vi "About Dialog.vi"(9 "E-mail:":string="msira@cmil.cz", 10 "Maintainer:":string="Martin Šíra", 11 "Title":string="Filter function meter - WAC software bundle") -> ()   [LabVIEW 2020]
doc: "Shows application about dialog."
uses:
  <vilib>/Platform/browser.llb/Open URL in Default Browser (string).vi
  external libraries/varilib/varilib.lvlib
panel:
  in  "open web":bool
  out "copyright":string="author"
  in  "OK":bool
  out "address":string="Created in scope of the EPM project WAC.\nDistributed under the MIT license.\n\nAuthors:\n Martin Šíra, msira@cmi.cz\n \n For authors of the low level instrument drivers see\n readmes in the sourcecode."
  out "www:":string="http://www.tracepqm.cmi.cz\nhttps://github.com/smaslan/TWM"
  out "Version:":string
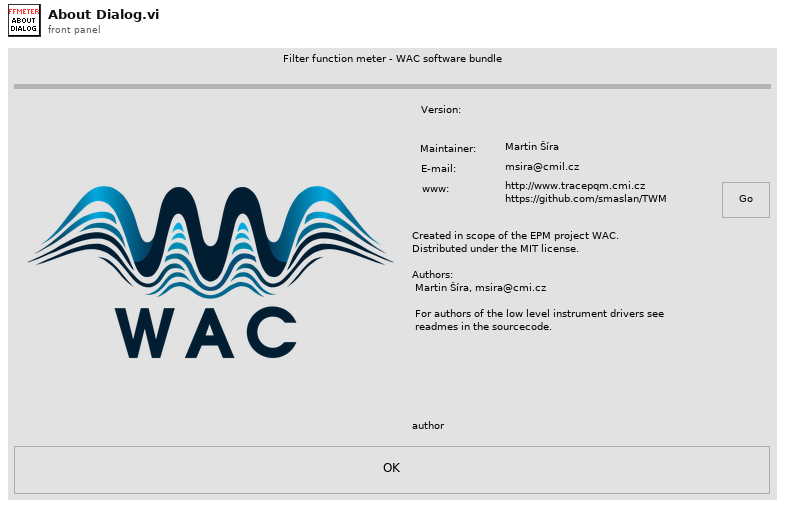
[diagram p1: front panel]
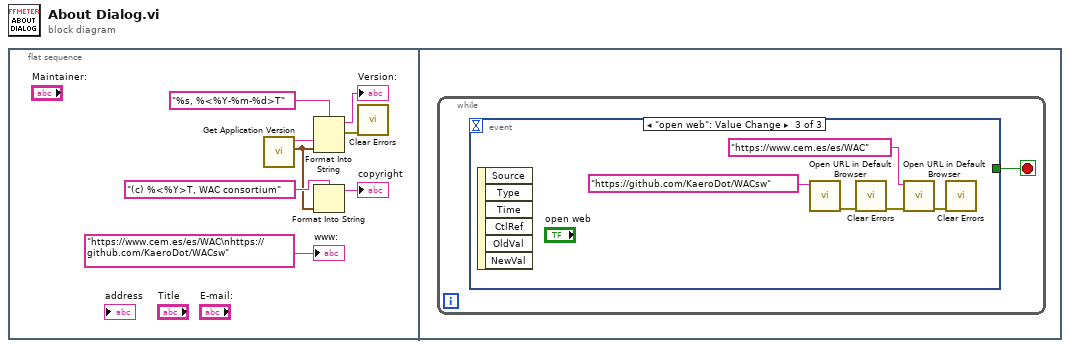
[diagram p0: block diagram]
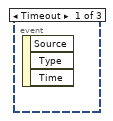
[diagram p2: hidden frame]
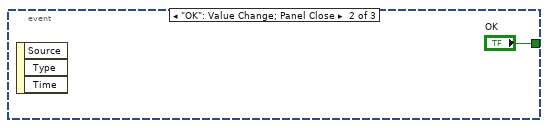
[diagram p3: hidden frame]
diagram:
  n1 = flat-sequence {
    frame #0 {
      n2 = call "Get Application Version.vi"() -> ("exe file last modification"=w1:timestamp, "version number sentence"=w2:string)  [unwired: 8 in, 2 out]
      n3 = Format Into String(format string="%s, %<%Y-%m-%d>T" ("time format string (%c)"), w2, w1) -> (resulting string=→"Version:":string, error out=w7:errorcluster)  [unwired: 2 in]
      n4 = Format Into String(format string="(c) %<%Y>T, WAC consortium", w1) -> (resulting string=→"copyright":string)  [unwired: 2 in, 1 out]
      n5 = call <vilib>:"Clear Errors.vi"("error in (no error)"=w7) -> ()  [unwired: 5 in, 2 out]
      "www:" <- "https://www.cem.es/es/WAC\nhttps://github.com/KaeroDot/WACsw" ("URL")
    }
    frame #1 {
      n6 = while {
        stop <- w9 stop-if-true
        n7 = event shown="[2] \"open web\": Value Change" {
          selector: _ -> [_ _ _]
          dyn-events: _ -> [_ _ _]
          timeout: _ -> [_ _ _]
          tunnel: [_ "OK" _] -> w9
          event Timeout {
            n8 = event-data() -> ()  [unwired: 1 in, 3 out]
          }
          event "OK": Value Change; Panel Close {
            n9 = event-data() -> ()  [unwired: 1 in, 3 out]
          }
          event "open web": Value Change {
            n10 = event-data() -> ()  [unwired: 1 in, 6 out]
            n11 = call-poly <vilib>:"Open URL in Default Browser.vi"("URL"="https://github.com/KaeroDot/WACsw") -> ("error out"=w14:errorcluster)  [unwired: 5 in, 1 out]
            n12 = call <vilib>:"Clear Errors.vi"("error in (no error)"=w14) -> ("error out"=w13:errorcluster)  [unwired: 5 in, 1 out]
            n13 = call-poly <vilib>:"Open URL in Default Browser.vi"("error in (no error)"=w13, "URL"="https://www.cem.es/es/WAC") -> ("error out"=w15:errorcluster)  [unwired: 4 in, 1 out]
            n14 = call <vilib>:"Clear Errors.vi"("error in (no error)"=w15) -> ()  [unwired: 5 in, 2 out]
          }
        }
      }
    }
  }
